vi "create distribution plot.vi"(4 "y bin":i32=100, 5 "y row":i32=4, 6 "x bin":i32=100, 7 "x row":i32=3, 8 "error in (no error)":errorcluster, 9 "length":i32, 10 "start":i32, 11 "Path":path=path "C:/Users/yg/Desktop/tmp/20230314-220729 s21time.dat") -> (0 "error out":errorcluster, 2 "Cluster":T1, 3 "Intensity Graph":dbl[][](graph))   [LabVIEW 2021]
uses:
  <vilib>/Utility/file.llb/Read Delimited Spreadsheet (DBL).vi
panel:
  # "If Length is zero, assume full data"
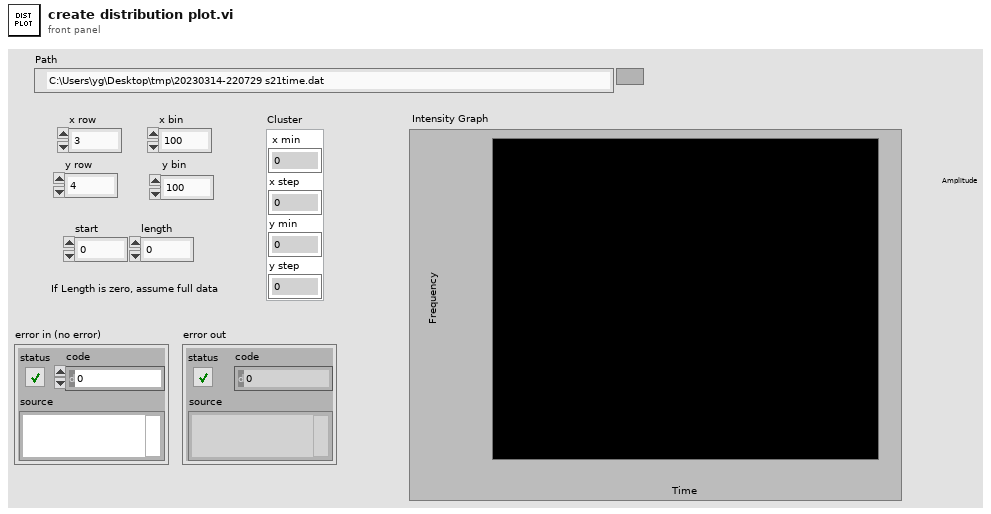
[diagram p1: front panel]
types:
  T1 = cluster{" x min":dbl, "x step":dbl, "y min":dbl, "y step":dbl}
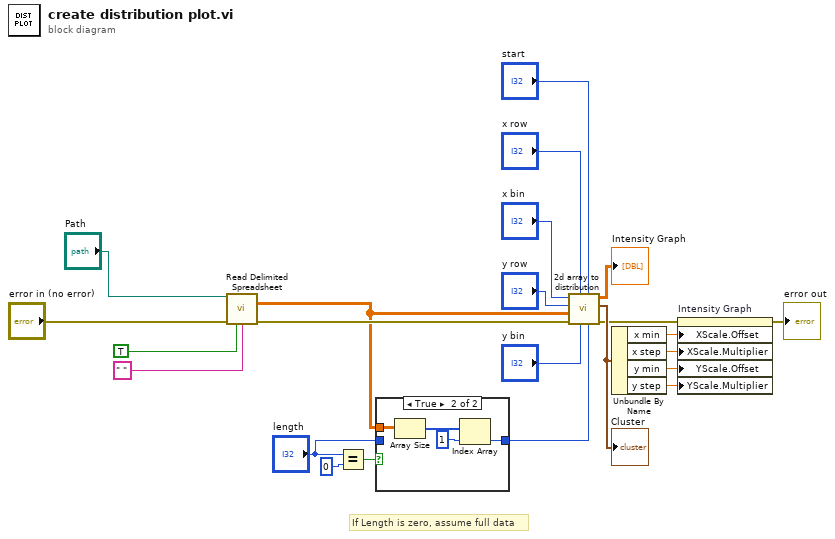
[diagram p0: block diagram]
diagram:
  # "If Length is zero, assume full data"
  n1 = call-poly <vilib>:"Read Delimited Spreadsheet.vi"("file path (dialog if empty)"="Path", "error in (no error)"="error in (no error)", "transpose? (F)"=TRUE, "delimiter (\\t)"=" " ("delimiter (\\t)")) -> ("all rows"=w1:dbl[][], "error out"=w8:errorcluster)  [unwired: 6 in, 4 out]
  n2 = Equal?(x="length", y=0) -> (x = y?=w4:bool)
  n3 = case shown="True" w4 {
    tunnel: [w24 w26] -> w3
    tunnel: "length" -> [w24 _]
    tunnel: w1 -> [_ w28]
    frame False {
    }
    frame True {
      n4 = Array Size(array=w28) -> (size(s)=w27:i32[])
      n5 = Index Array(array=w27, index=1) -> (element=w26:i32)
    }
  }
  n6 = call "2d array to distribution.vi"("length"=w3, "start"="start", "y bin"="y bin", "x row"="x row", "error in (no error)"=w8, "all rows"=w1, "y row"="y row", "x bin"="x bin") -> ("error out"=w7:errorcluster, "Cluster"=w14:T1, "Array"=→"Intensity Graph":dbl[][])  [unwired: 1 in]
  "Cluster" <- w14
  n7 = Unbundle By Name(w14) -> ("x min"=w13:dbl, "x step"=w12:dbl, "y min"=w11:dbl, "y step"=w10:dbl)
  n8 = property on="Intensity Graph" class="IntGraph (strict)"(error in=w7, "XScale.Offset"=w13, "XScale.Multiplier"=w12, "YScale.Offset"=w11, "YScale.Multiplier"=w10) -> (error out=→"error out":errorcluster)  [unwired: 1 in, 1 out]
